vi "Read.vi"(8 "error in (no error)":errorcluster, 9 "Variant":variant, 11 "UDP in":refnum<class "UDP.lvclass">) -> (0 "error out":errorcluster, 2 "String":string, 3 "UDP out":refnum<class "UDP.lvclass">)   [LabVIEW 2023, in "Protocols.lvlib" / "UDP.lvclass"]
uses:
  UDP.lvclass
  Protocol Parent/Methods/Read Parameter.ctl
  Protocol Parent/Protocol Parent.lvclass
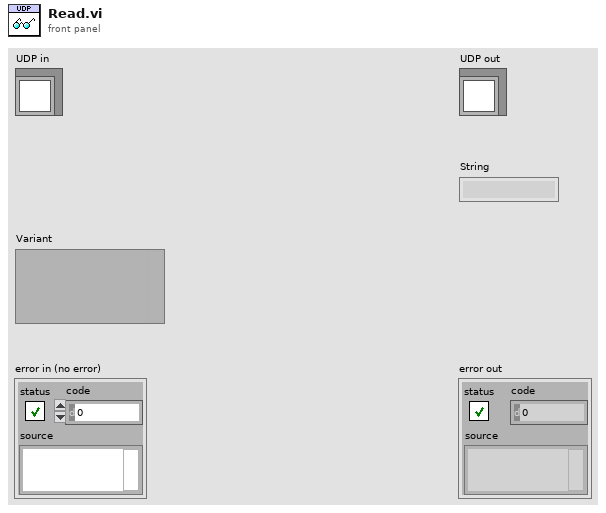
[diagram p1: front panel]
types:
  T1 = typedef "Protocols.lvlib/Protocol Parent.lvclass/Read Parameter.ctl" = cluster{"Wait Type":enum16{"Byte Count", "Wait sec"}, "Wait Value":dbl}
  T2 = enum16{"Standard", "Buffered", "CRLF", "Immediate"}
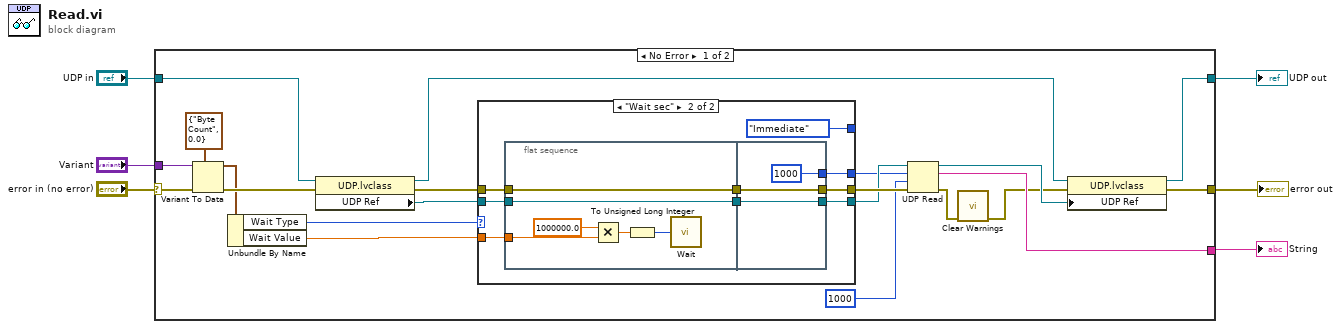
[diagram p0: block diagram]
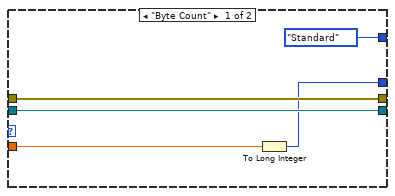
[diagram p2: hidden frame]
diagram:
  n1 = case shown="No Error" "error in (no error)" {
    selector: "error in (no error)" -> [w22 w52]
    tunnel: "UDP in" -> [w27 w51]
    tunnel: [w25 w52] -> w3
    tunnel: [w23 w51] -> w1
    tunnel: "Variant" -> [w20 _]
    tunnel: [w13 _] -> w2
    frame No Error {
      n2 = Variant To Data(error in=w22, type=T1 {"Wait Type"=enum."Byte Count", "Wait Value"=0.0} ("Read Parameter"), Variant=w20) -> (data=w19:T1, error out=w21:errorcluster)
      n3 = Unbundle By Name(w19) -> ("Wait Type"=w15:enum16{"Byte Count", "Wait sec"}, "Wait Value"=w14:dbl)
      n4 = property class="UDP.lvclass"(reference=w27, error in=w21) -> (reference out=w24:refnum<class "UDP.lvclass">, error out=w18:errorcluster, "UDP Ref"=w17:refnum<k16>)
      n5 = case shown="\"Wait sec\"" w15 {
        tunnel: w18 -> [w32 w41]
        tunnel: w17 -> [w30 w40]
        tunnel: [w32 w39] -> w16
        tunnel: [w30 w38] -> w10
        tunnel: [w28 w34] -> w9
        tunnel: w14 -> [w31 w35]
        tunnel: [T2."Standard" ("mode (standard)") T2."Immediate" ("mode (standard)")] -> _
        frame "Byte Count" {
          n6 = To Long Integer(number=w31) -> (32bit integer=w28:i32)
        }
        frame "Wait sec" {
          n7 = flat-sequence {
            tunnel: w40 -> [w46]
            tunnel: w41 -> [w47]
            tunnel: [w47] -> w37
            tunnel: [w46] -> w36
            tunnel: w35 -> [w45]
            tunnel: [w50] -> w39
            tunnel: [w49] -> w38
            tunnel: w37 -> [w50]
            tunnel: w36 -> [w49]
            tunnel: [1000 ("Wait Value")] -> w34
            frame #0 {
              n8 = Multiply(x=1000000.0, y=w45) -> (x*y=w44:dbl)
              n9 = To Unsigned Long Integer(number=w44) -> (unsigned 32bit integer=w42:u32)
              n10 = call "Wait"("Count(uSec)"=w42) -> ()  [unwired: 1 out]
            }
            frame #1 {
            }
          }
        }
      }
      n11 = UDP Read(connection ID=w10, max size (548)=w9, timeout ms (25000)=1000, 8:w16) -> (data out=w13:string, error out=w8:errorcluster, 3:w26:refnum<k16>)  [unwired: 2 out]
      n12 = call "Clear Warnings.vi"("error in (no error)"=w8) -> ("error out"=w7:errorcluster)  [unwired: 10 in]
      n13 = property class="UDP.lvclass"(reference=w24, error in=w7, "UDP Ref"=w26) -> (reference out=w23:refnum<class "UDP.lvclass">, error out=w25:errorcluster)
    }
    frame Error {
    }
  }
  "error out" <- w3
  "UDP out" <- w1
  "String" <- w2
